vi "Values from States.vi"(10 "Desired\nState":i32, 11 "Current\nState":i32 min=0 max=6) -> (0 "Enable Elbow\nBrake":bool=TRUE, 1 "Enable Shoulder\nBrake":bool=TRUE, 2 "Change in\nElbow Angle":dbl, 3 "Change in\nShoulder Angle":dbl)   [LabVIEW 2017]
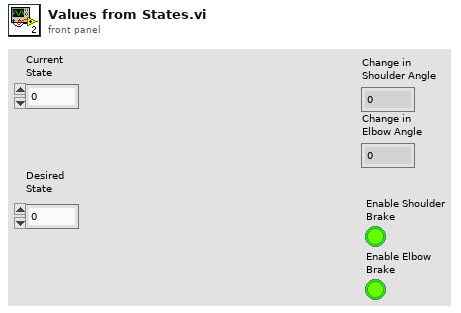
[diagram p1: front panel]
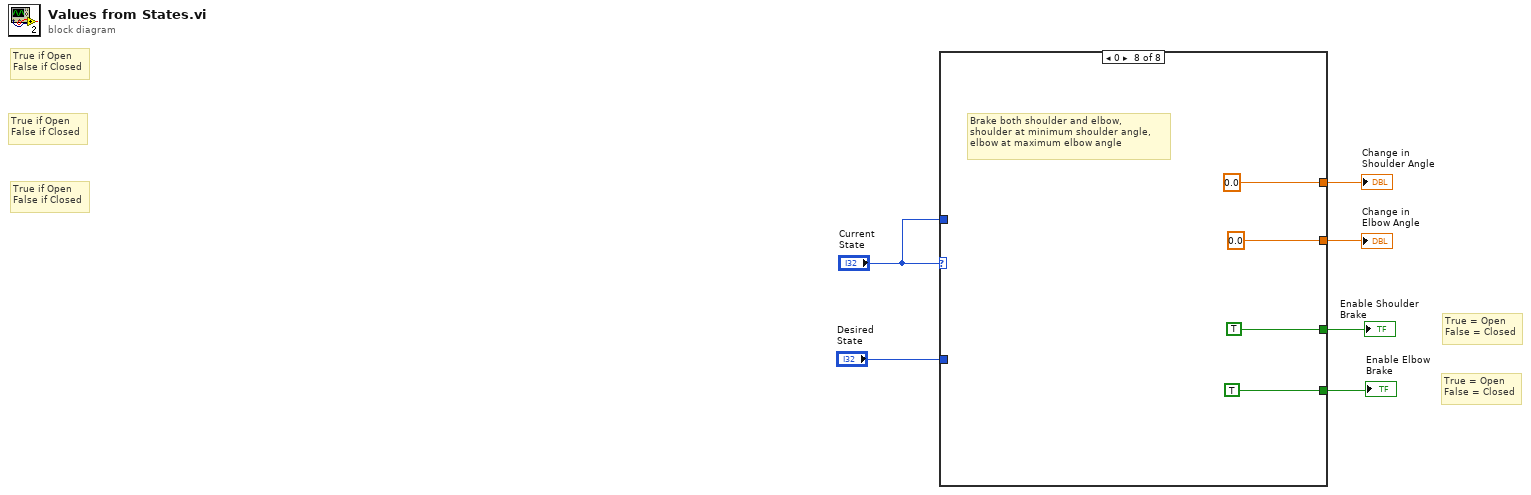
[diagram p0: block diagram]
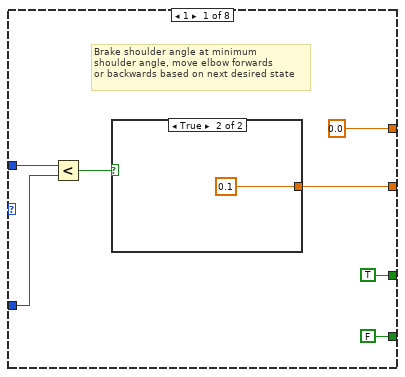
[diagram p2: hidden frame]
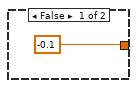
[diagram p3: hidden frame]
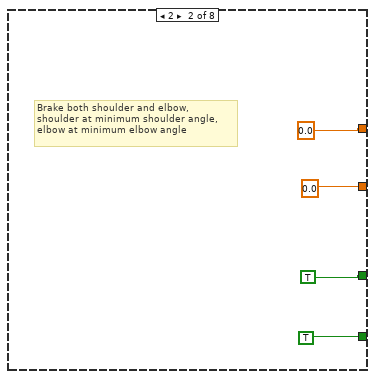
[diagram p4: hidden frame]
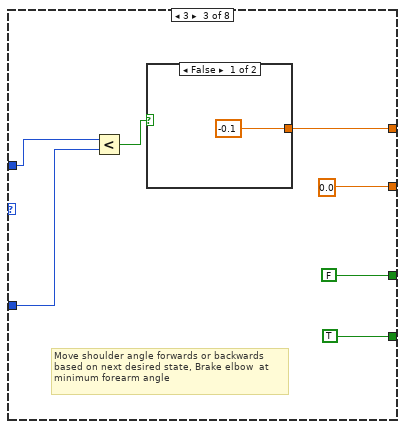
[diagram p5: hidden frame]
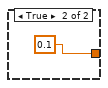
[diagram p6: hidden frame]
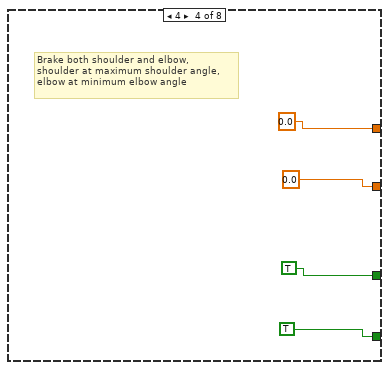
[diagram p7: hidden frame]
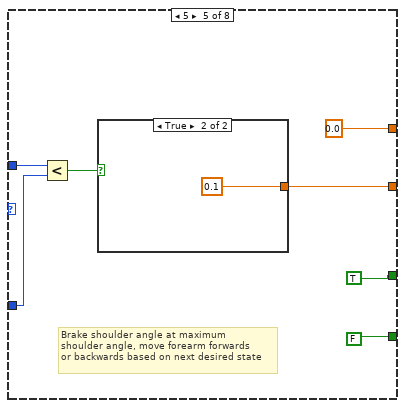
[diagram p8: hidden frame]
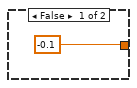
[diagram p9: hidden frame]
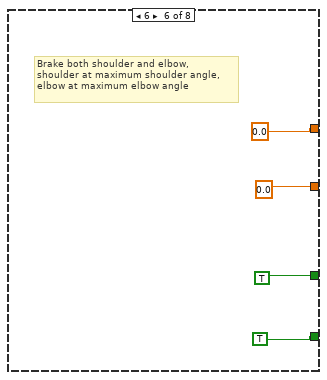
[diagram p10: hidden frame]
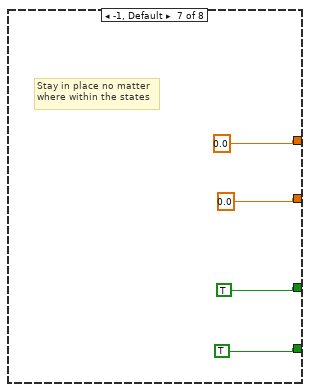
[diagram p11: hidden frame]
diagram:
  # "True = Open\nFalse = Closed"
  # "True = Open\nFalse = Closed"
  # "True if Open\nFalse if Closed"
  # "True if Open\nFalse if Closed"
  # "True if Open\nFalse if Closed"
  n1 = case shown="0" "Current\nState" {
    tunnel: [TRUE TRUE FALSE TRUE TRUE TRUE TRUE TRUE] -> w6
    tunnel: [FALSE TRUE TRUE TRUE FALSE TRUE TRUE TRUE] -> w5
    tunnel: [w9 0.0 ("Change in\nElbow Angle") 0.0 ("Change in\nElbow Angle") 0.0 ("Change in\nElbow Angle") w33 0.0 ("Change in\nElbow Angle") 0.0 ("Change in\nElbow Angle") 0.0 ("Change in\nElbow Angle")] -> w4
    tunnel: [0.0 ("Change in\nElbow Angle") 0.0 ("Change in\nElbow Angle") w20 0.0 ("Change in\nElbow Angle") 0.0 ("Change in\nElbow Angle") 0.0 ("Change in\nElbow Angle") 0.0 ("Change in\nElbow Angle") 0.0 ("Change in\nElbow Angle")] -> w3
    tunnel: "Desired\nState" -> [w13 _ w25 _ w37 _ _ _]
    tunnel: "Current\nState" -> [w12 _ w26 _ w38 _ _ _]
    frame 1 {
      # "Brake shoulder angle at minimum\nshoulder angle, move elbow forwards\nor backwards based on next desired state"
      n2 = Less?(x=w12, y=w13) -> (x < y?=w11:bool)
      n3 = case shown="True" w11 {
        tunnel: [-0.1 ("Change in\nElbow Angle") 0.1 ("Change in\nElbow Angle")] -> w9
        frame False {
        }
        frame True {
        }
      }
    }
    frame 2 {
      # "Brake both shoulder and elbow,\nshoulder at minimum shoulder angle,\nelbow at minimum elbow angle"
    }
    frame 3 {
      # "Move shoulder angle forwards or backwards\nbased on next desired state, Brake elbow  at\nminimum forearm angle"
      n4 = Less?(x=w26, y=w25) -> (x < y?=w21:bool)
      n5 = case shown="False" w21 {
        tunnel: [-0.1 0.1] -> w20
        frame False {
        }
        frame True {
        }
      }
    }
    frame 4 {
      # "Brake both shoulder and elbow,\nshoulder at maximum shoulder angle,\nelbow at minimum elbow angle"
    }
    frame 5 {
      # "Brake shoulder angle at maximum\nshoulder angle, move forearm forwards\nor backwards based on next desired state"
      n6 = Less?(x=w38, y=w37) -> (x < y?=w39:bool)
      n7 = case shown="True" w39 {
        tunnel: [-0.1 ("Change in\nElbow Angle") 0.1 ("Change in\nElbow Angle")] -> w33
        frame False {
        }
        frame True {
        }
      }
    }
    frame 6 {
      # "Brake both shoulder and elbow,\nshoulder at maximum shoulder angle,\nelbow at maximum elbow angle"
    }
    frame -1, Default {
      # "Stay in place no matter\nwhere within the states"
    }
    frame 0 {
      # "Brake both shoulder and elbow,\nshoulder at minimum shoulder angle,\nelbow at maximum elbow angle"
    }
  }
  "Change in\nShoulder Angle" <- w3
  "Change in\nElbow Angle" <- w4
  "Enable Shoulder\nBrake" <- w6
  "Enable Elbow\nBrake" <- w5
